vi "Build Region.vi"(11 "Plant Positions":map{T1, u32}(c390)) -> (3 "Plant Regions":map{T1, u32}[](array[numeric]))   [LabVIEW 2024]
uses:
  Utility/Universal Utility/TypeDefs_Utility/Cluster_Row-Column.ctl
  Utility/Universal Utility/TypeDefs_Utility/ENUM_4 Directions U-D-L-R.ctl
  1ac3296f-e1bc-4bd6-9de7-9b5db7959bee.vi
  1ac3296f-e1bc-4bd6-9de7-9b5db7959bee.vi/0a5f5d0f-6921-449f-9499-5f6c7f3eae0e.vi
  1ac3296f-e1bc-4bd6-9de7-9b5db7959bee.vi/2f57c213-34d0-4fb8-93c4-9da21d141025.vi
  <vilib>/Utility/error.llb/Trim Whitespace.vi
  <vilib>/Utility/error.llb/Trim Whitespace One-Sided.vi
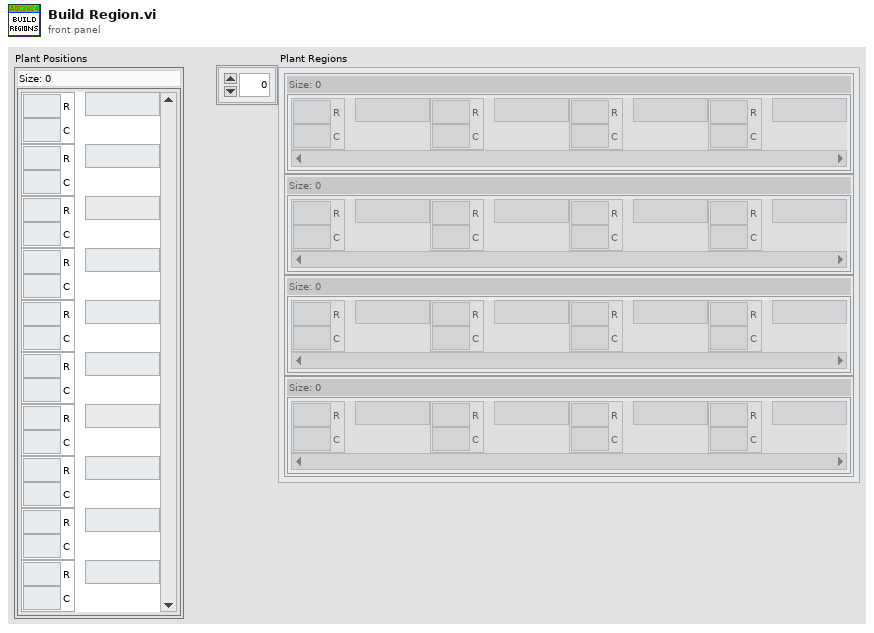
[diagram p1: front panel]
types:
  T1 = typedef "Cluster_Row-Column.ctl" = cluster{"R":i32, "C":i32}
  T2 = typedef "ENUM_4 Directions U-D-L-R.ctl" = enum16{"Up;-1,0", "Right;0,1", "Down;1,0", "Left;0,-1"}
  T3 = typedef "Cluster_X-Y.ctl" = cluster{"X":u64, "Y":u64}
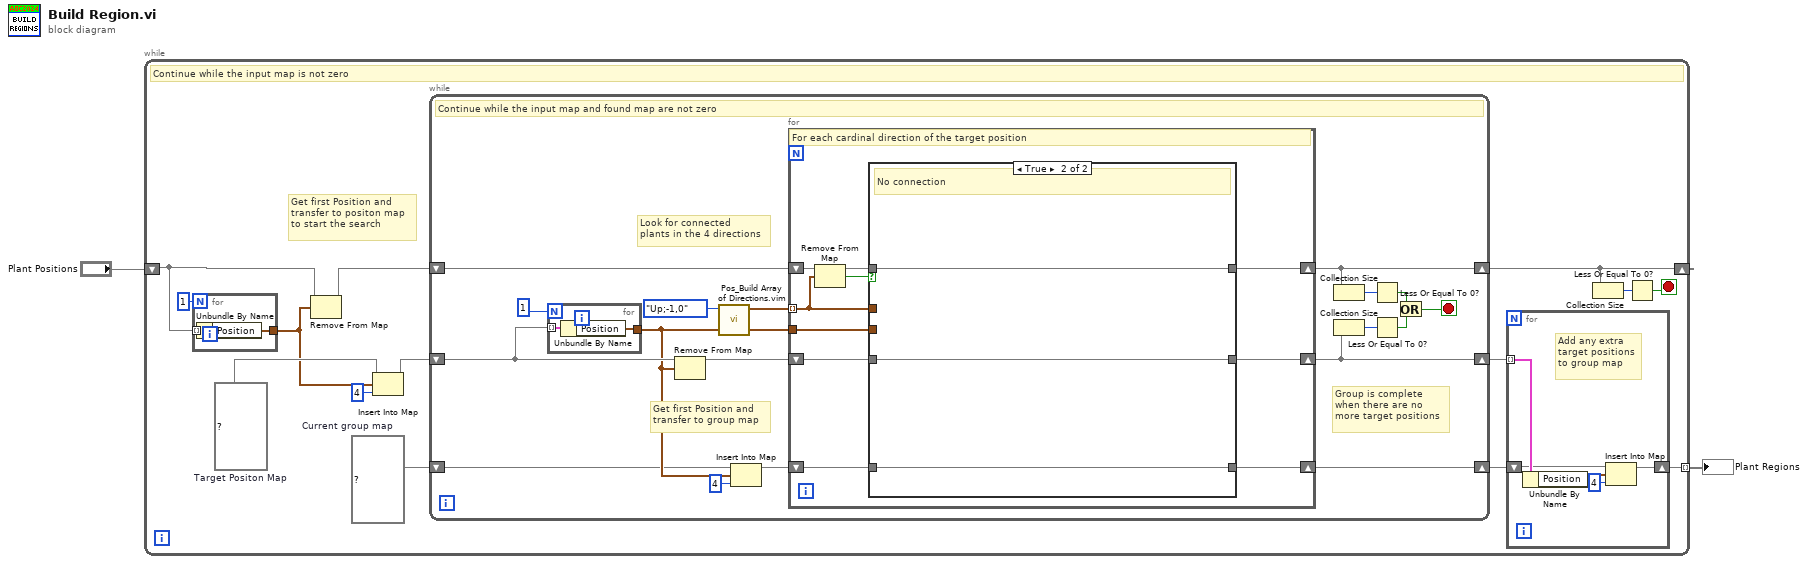
[diagram p0: block diagram]
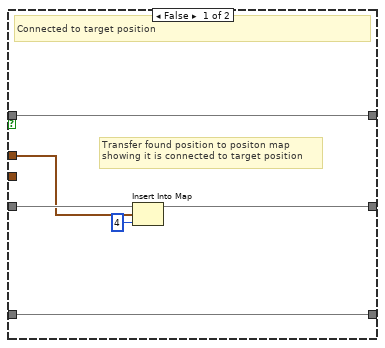
[diagram p2: hidden frame]
diagram:
  n1 = while {
    shift-right: [w14] -> _
    shift-left: "Plant Positions" -> [w12]
    tunnel: [w4] -> w2 mode=indexing
    stop <- w15 stop-if-true
    w7 = map{T1, u32} {}  # Current group map
    w10 = map{T1, u32} {}  # Target Positon Map
    # "Get first Position and\ntransfer to positon map\nto start the search"
    # "Continue while the input map is not zero"
    n2 = for {
      N: 1 -> [_]
      tunnel: w12 -> [w23] mode=indexing
      tunnel: [w22] -> w8
      n3 = Unbundle By Name(w23) -> ("Position"=w22:T1)
    }
    n4 = Remove From Map(10:w8, 11:w12) -> (3:w11:map{T1, u32})  [unwired: 2 out]
    n5 = Insert Into Map(map in=w10, key=w8, value=u32 4) -> (map out=w9:map{T1, u32})  [unwired: 2 out]
    n6 = while {
      shift-right: [w38] -> w14
      shift-left: w11 -> [w40]
      shift-right: [w36] -> w6
      shift-left: w9 -> [w30]
      shift-right: [w26] -> w5
      shift-left: w7 -> [w25]
      stop <- w32 stop-if-true
      # "Group is complete\nwhen there are no\nmore target positions"
      # "Look for connected \nplants in the 4 directions"
      # "Get first Position and\ntransfer to group map"
      # "Continue while the input map and found map are not zero"
      n7 = for {
        N: 1 -> [_]
        tunnel: w30 -> [w43] mode=indexing
        tunnel: [w42] -> w28
        n8 = Unbundle By Name(w43) -> ("Position"=w42:T1)
      }
      n9 = Remove From Map(10:w28, 11:w30) -> (3:w29:map{T1, u32})  [unwired: 2 out]
      n10 = call "Pos_Build Array of Directions.vim"("Positon"=w28, "Direction"=ENUM_4_Directions_U-D-L-R."Up;-1,0") -> ("Direction Positions Out"=w39:T3[])  [unwired: 9 in]
      n11 = Insert Into Map(map in=w25, key=w28, value=u32 4) -> (map out=w27:map{T1, u32})  [unwired: 2 out]
      n12 = for {
        shift-right: [w51] -> w36
        shift-left: w29 -> [w53]
        shift-right: [w52] -> w38
        shift-left: w40 -> [w49]
        tunnel: w39 -> [w45] mode=indexing
        tunnel: w28 -> [w47]
        shift-right: [w44] -> w26
        shift-left: w27 -> [w46]
        # "For each cardinal direction of the target position"
        n13 = Remove From Map(10:w45, 11:w49) -> (2:w50:bool, 3:w48:map{T1, u32})  [unwired: 1 out]
        n14 = case shown="True" w50 {
          tunnel: w48 -> [w56 w62]
          tunnel: w53 -> [w59 w61]
          tunnel: [w56 w62] -> w52
          tunnel: [w58 w61] -> w51
          tunnel: w47 -> [_ _]
          tunnel: w46 -> [w54 w60]
          tunnel: w45 -> [w57 _]
          tunnel: [w54 w60] -> w44
          frame False {
            # "Transfer found position to positon map\nshowing it is connected to target position"
            # "Connected to target position"
            n15 = Insert Into Map(map in=w59, key=w57, value=u32 4) -> (map out=w58:map{T1, u32})  [unwired: 2 out]
          }
          frame True {
            # "No connection"
          }
        }
      }
      n16 = Collection Size(1:w38) -> (0:w37:i32)
      n17 = Collection Size(1:w36) -> (0:w35:i32)
      n18 = Less Or Equal To 0?(x=w37) -> (x <= 0?=w34:bool)
      n19 = Less Or Equal To 0?(x=w35) -> (x <= 0?=w33:bool)
      n20 = Or(x=w34, y=w33) -> (x .or. y?=w32:bool)
    }
    n21 = for {
      tunnel: w6 -> [w21] mode=indexing
      shift-right: [w19] -> w4
      shift-left: w5 -> [w20]
      # "Add any extra\ntarget positions\nto group map"
      n22 = Unbundle By Name(w21) -> ("Position"=w18:T1)
      n23 = Insert Into Map(map in=w20, key=w18, value=u32 4) -> (map out=w19:map{T1, u32})  [unwired: 2 out]
    }
    n24 = Collection Size(1:w14) -> (0:w16:i32)
    n25 = Less Or Equal To 0?(x=w16) -> (x <= 0?=w15:bool)
  }
  "Plant Regions" <- w2
